vi "deleteVariable.vi"(0 "Variable Manager Trigger Event":refnum<class "HGF_Event.lvclass">, 2 "Shared Variable":refnum<k21>, 3 "timeout":i32, 5 "error in (no error)":errorcluster) -> (16 "delete Variable timed out":bool, 19 "error out":errorcluster)   [LabVIEW 2009, in "MoAgSy.lvlib"]
uses:
  MoAgSy.lvlib
  HGF_BaseClasses/HGF_Event/HGF_Event.lvclass
  HGF_SV/HGF_SVFactory/HGF_SVFactory.lvclass
  HGF_BaseClasses/HGF_TriggeredEvent/HGF_TriggeredEvent.lvclass
  HGF_SV/Visitors/HGF_SVVarManVisitor_delete/HGF_SVVarManVisitor_delete.lvclass
  HGF_BaseClasses/HGF_Factory/HGF_Factory.lvclass
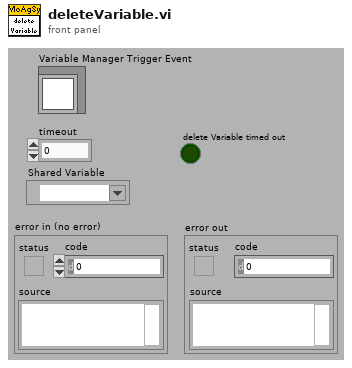
[diagram p1: front panel]
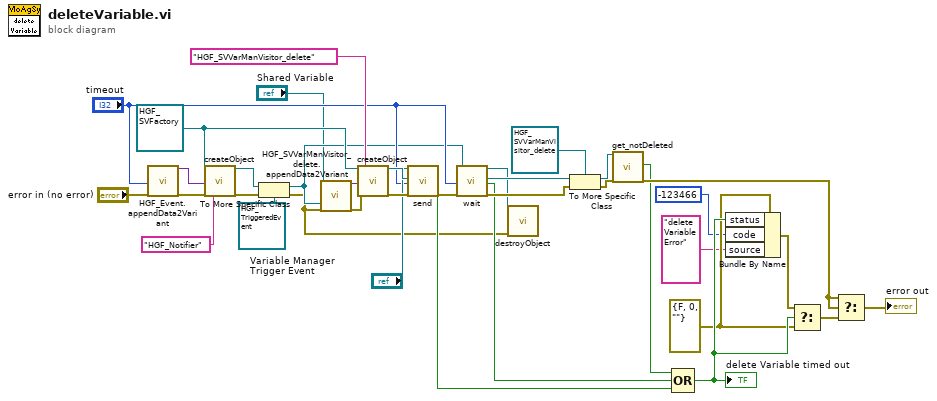
[diagram p0: block diagram]
diagram:
  w14 = errorcluster {"status"=FALSE, "code"=0, "source"=""} ("error out")
  w28 = refnum<class "HGF_SVFactory.lvclass"> refnum ("HGF_SV.lvlib:HGF_SVFactory.lvclass")
  n1 = call "HGF_Event.appendData2Variant.vi"("timeout in ms (-1)"="timeout", "error in (no error)"="error in (no error)") -> ("dup initData"=w30:variant, "error out"=w29:errorcluster)  [unwired: 16 in]
  n2 = call "createObject.vi"("HGF_Factory"=w28, "initializationData"=w30, "error in (no error)"=w29, "className"="HGF_Notifier") -> ("HGF_Object"=w25:refnum<class "HGF_Factory.lvclass">, "error out"=w23:errorcluster)  [unwired: 1 in, 13 out]
  n3 = To More Specific Class(target class=refnum<class "HGF_TriggeredEvent.lvclass"> refnum ("DSC Exception"), reference=w25, error in=w23) -> (specific class reference=w9:refnum<class "HGF_TriggeredEvent.lvclass">, error out=w7:errorcluster)
  n4 = call "HGF_SVVarManVisitor_delete.appendData2Variant.vi"("Shared Variable"="Shared Variable", "return-to Event"=w9, "error in"=w7) -> ("dup variant"=w10:variant, "error out"=w6:errorcluster)  [unwired: 15 in]
  n5 = call "createObject.vi"("HGF_Factory"=w28, "initializationData"=w10, "error in (no error)"=w6, "className"="HGF_SVVarManVisitor_delete") -> ("HGF_Object"=w22:refnum<class "HGF_Factory.lvclass">, "error out"=w21:errorcluster)  [unwired: 1 in, 13 out]
  n6 = call-dynamic "send.vi"("HGF_Event"="Variable Manager Trigger Event", "Object"=w22, "timeout in ms (-1)"="timeout", "error in (no error)"=w21) -> ("timed out?"=w35:bool, "error out"=w20:errorcluster)  [unwired: 13 in, 1 out]
  n7 = call-dynamic "wait.vi"("HGF_Event"=w9, "msTimeout (-1)"="timeout", "error in (no error)"=w20) -> ("dup HGF_Event"=w15:refnum<class "HGF_TriggeredEvent.lvclass">, "Object"=w17:refnum<class>, "timed out"=w13:bool, "error out"=w16:errorcluster)  [unwired: 13 in]
  n8 = call "destroyObject.vi"("HGF_Factory"=w15, "error in (no error)"=w7) -> ()  [unwired: 17 in, 1 out]
  n9 = To More Specific Class(target class=refnum<class "HGF_SVVarManVisitor_delete.lvclass"> refnum ("HGF_SV.lvlib:HGF_SVVarManVisitor_delete.lvclass"), reference=w17, error in=w16) -> (specific class reference=w5:refnum<class "HGF_SVVarManVisitor_delete.lvclass">, error out=w3:errorcluster)
  n10 = call "get_notDeleted.vi"("HGF_SVVarManVisitor_delete"=w5, "error in (no error)"=w3) -> ("not deleted?"=w1:bool, "error out"=w2:errorcluster)  [unwired: 15 in, 1 out]
  n11 = Compound Arithmetic op=OR(w1, w13, w35) -> (w34:bool)
  "delete Variable timed out" <- w34
  n12 = Bundle By Name(cluster=w14, "status"=w34, "code"=-123466, "source"="delete Variable Error") -> (w31:errorcluster)
  n13 = Select(t=w31, s=w34, f=w14) -> (s? t:f=w32:errorcluster)
  n14 = Select(t=w2, s=w2, f=w32) -> (s? t:f=→"error out":errorcluster)
